vi "Shooter Main.vi"   [LabVIEW 2017]
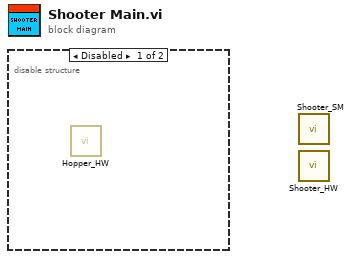
[diagram p0: block diagram]
diagram:
  n1 = disable-structure shown="Disabled" {
    frame Disabled {
      n2 = call "Hopper_HW.vi"() -> ()  [unwired: 12 in]
    }
    frame Enabled {
    }
  }
  n3 = call "Shooter_SM.vi"() -> ()  [unwired: 12 in]
  n4 = call "Shooter_HW.vi"() -> ()  [unwired: 12 in]
